vi "OSC reverse converter.vi"(1 "2D OSC Configuration":T2(array[cluster])) -> (0 "1D OSC Configuration":T1(array[cluster]))   [LabVIEW 2013]
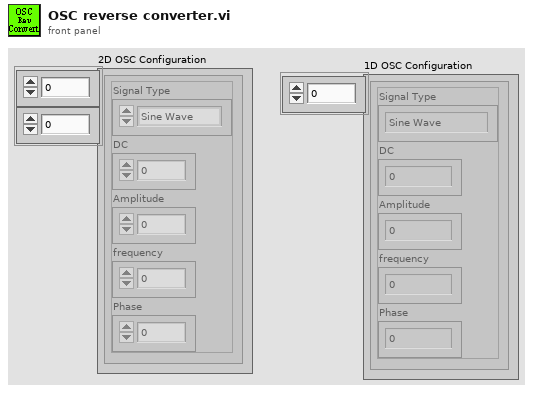
[diagram p1: front panel]
types:
  T1 = cluster{"Signal Type":enum16{"Sine Wave", "Triangle Wave", "Square Wave", "Sawtooth Wave"}, "DC":dbl, "Amplitude":dbl, "frequency":dbl, "Phase":dbl}[]
  T2 = cluster{"Signal Type":enum16{"Sine Wave", "Triangle Wave", "Square Wave", "Sawtooth Wave"}, "DC":dbl, "Amplitude":dbl, "frequency":dbl, "Phase":dbl}[][]
  T3 = cluster{"Signal Type":enum16{"Sine Wave", "Triangle Wave", "Square Wave", "Sawtooth Wave"}, "DC":dbl, "Amplitude":dbl, "frequency":dbl, "Phase":dbl}
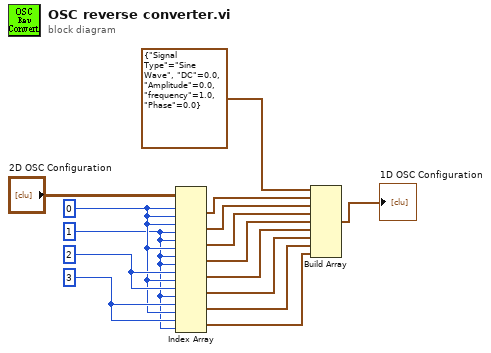
[diagram p0: block diagram]
diagram:
  w13 = 3
  w14 = 2
  w11 = 1
  w12 = 0
  n1 = Index Array(array="2D OSC Configuration", index (row) #1=w12, index (col) #1=w12, index (row) #2=w12, index (col) #2=w11, index (row) #3=w11, index (col) #3=w12, index (row) #4=w11, index (col) #4=w11, index (row) #5=w14, index (col) #5=w12, index (row) #6=w14, index (col) #6=w11, index (row) #7=w13, index (col) #7=w12, index (row) #8=w13, index (col) #8=w11) -> (element #1=w10:T3, element #2=w9:T3, element #3=w8:T3, element #4=w7:T3, element #5=w6:T3, element #6=w5:T3, element #7=w4:T3, element #8=w3:T3)
  n2 = Build Array(T3 {"Signal Type"=enum."Sine Wave", "DC"=0.0, "Amplitude"=0.0, "frequency"=1.0, "Phase"=0.0} ("Default OSC"), w10, w9, w8, w7, w6, w5, w4, w3) -> (→"1D OSC Configuration":T1)
